vi "Wait for Initialized.vi"(0 "Refnum in":refnum<k20>, 11 "error in (no error)":errorcluster) -> (4 "Refnum out":refnum<k20>, 6 "CLIP state":T1, 15 "error out":errorcluster)   [LabVIEW 2020, in "My Network Host v1.lvlib"]
uses:
  My Network Host v1.lvlib
  <vilib>/Utility/error.llb/Error Cluster From Error Code.vi
  <vilib>/rvi/errors/niLvFpgaAdjustHostInterfaceError.vi
  <vilib>/rvi/interface/nirviReadWriteControl/nirviReadWriteControl.xnode
  NiFpgaLv.dll
  <vilib>/rvi/interface/Simulation/niFpgaSimulationCallBeginRW.vi
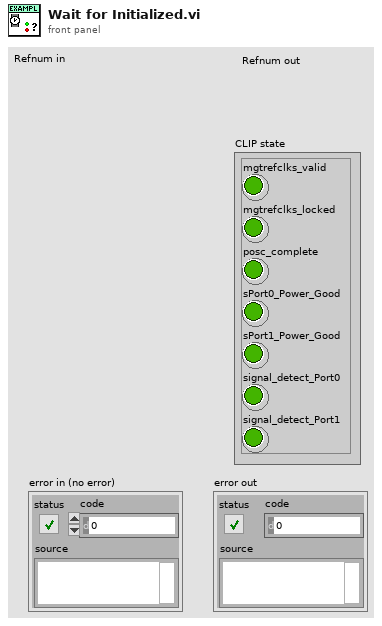
[diagram p1: front panel]
types:
  T1 = cluster{"mgtrefclks_valid":bool, "mgtrefclks_locked":bool, "posc_complete":bool, "sPort0_Power_Good":bool, "sPort1_Power_Good":bool, "signal_detect_Port0":bool, "signal_detect_Port1":bool}
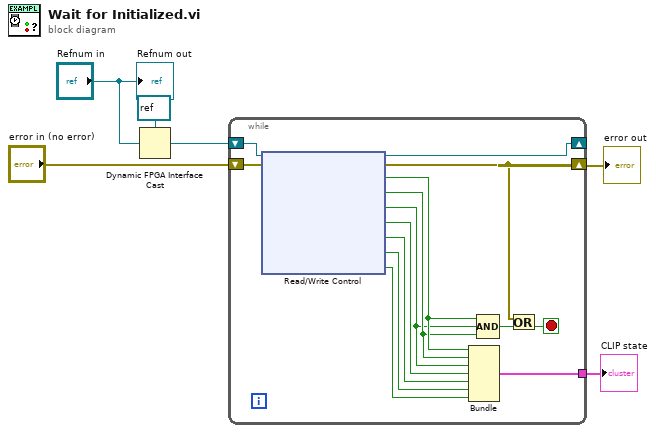
[diagram p0: block diagram]
diagram:
  n1 = Dynamic FPGA Interface Cast(Session In=refnum<k20> refnum ("Refnum in"), Type="Refnum in") -> (Session Out=w1:refnum<k20>)
  n2 = while {
    shift-right: [w19] -> _
    shift-left: w1 -> [w20]
    shift-right: [w15] -> w6
    shift-left: "error in (no error)" -> [w18]
    tunnel: [w7] -> w4
    stop <- w16 stop-if-true
    n3 = xnode "Read/Write Control"("FPGA VI Reference In"=w20, "error in"=w18) -> ("FPGA VI Reference Out"=w19:refnum<k20>, "error out"=w15:errorcluster, "mgtrefclks_valid"=w14:bool, "mgtrefclks_locked"=w13:bool, "posc_complete"=w12:bool, "sPort0_Power_Good"=w11:bool, "sPort1_Power_Good"=w10:bool, "signal_detect_Port0"=w9:bool, "signal_detect_Port1"=w8:bool)
    n4 = Bundle("mgtrefclks_valid"=w14, "mgtrefclks_locked"=w13, "posc_complete"=w12, "sPort0_Power_Good"=w11, "sPort1_Power_Good"=w10, "signal_detect_Port0"=w9, "signal_detect_Port1"=w8) -> (w7:T1)  [unwired: 1 in]
    n5 = Compound Arithmetic op=AND(w14, w12, w13) -> (w17:bool)
    n6 = Or(x=w15, y=w17) -> (x .or. y?=w16:bool)
  }
  "error out" <- w6
  "CLIP state" <- w4
  "Refnum out" <- "Refnum in"
